vi "Z_ReflectorPosition_CT.vi"(10 "ReflectorPosition":i32) -> (2 "Command":string)   [LabVIEW 2017]
uses:
  sobot structures/SoBot_CommandTypes.ctl
  sobot structures/Z_Command.ctl
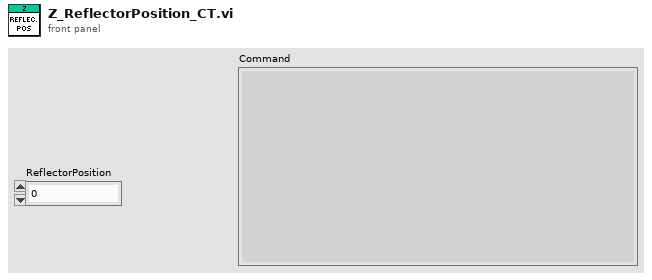
[diagram p1: front panel]
types:
  T1 = typedef "Z_Command.ctl" = enum16{"Z_Initialize", "Z_MoveToPosition", "Z_Focus", "Z_ReflectorPosition"}
  T2 = typedef "SoBot_CommandTypes.ctl" = enum16{"General_Command", "XY_Command", "Z_Command", "Plattform_Command"}
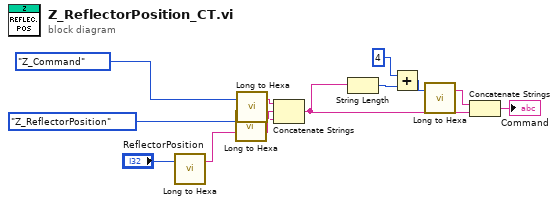
[diagram p0: block diagram]
diagram:
  n1 = call "Long to Hexa.vi"("Long"="ReflectorPosition") -> ("Hexa"=w3:string)  [unwired: 2 in]
  n2 = call "Long to Hexa.vi"("Long"=Z_Command."Z_ReflectorPosition" ("Z_Command")) -> ("Hexa"=w11:string)  [unwired: 2 in]
  n3 = call "Long to Hexa.vi"("Long"=SoBot_CommandTypes."Z_Command" ("SoBot_CommandTypes")) -> ("Hexa"=w12:string)  [unwired: 2 in]
  n4 = Concatenate Strings(w12, w11, w3) -> (w6:string)
  n5 = String Length(string=w6) -> (length=w10:i32)
  n6 = Add(x=4, y=w10) -> (x+y=w8:i32)
  n7 = call "Long to Hexa.vi"("Long"=w8) -> ("Hexa"=w7:string)  [unwired: 2 in]
  n8 = Concatenate Strings(w7, w6) -> (→"Command":string)
